vi "NML Bus Scan Sig Recovery 7265.vi"(3 "error in (no error)":errorcluster, 4 "String Read In":string, 5 "VISA Session":refnum<visa-resource-name>) -> (0 "error out":errorcluster, 1 "String Read Out":string, 2 "VISA Session Out":refnum<visa-resource-name>)   [LabVIEW 2021]
uses:
  <vilib>/regexp/Match Regular Expression.xnode
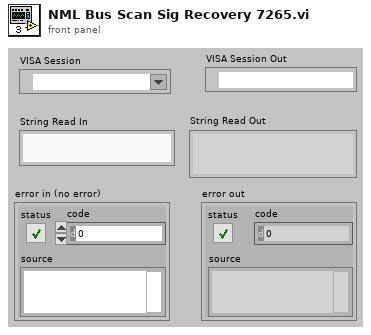
[diagram p1: front panel]
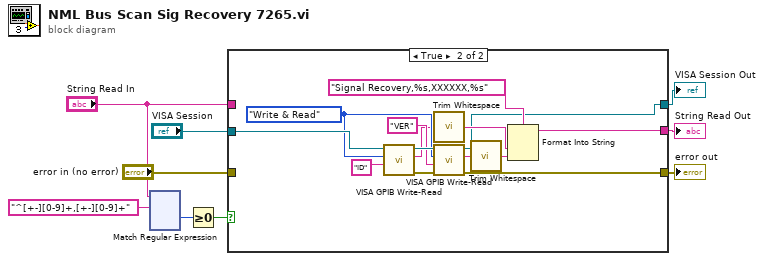
[diagram p0: block diagram]
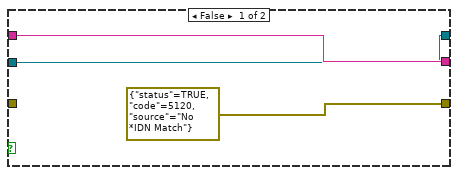
[diagram p2: hidden frame]
diagram:
  n1 = xnode "Match Regular Expression"("input string"="String Read In", "regular expression"="^[+-][0-9]+,[+-][0-9]+") -> ("offset past match"=w4:i32)  [unwired: 4 in, 4 out]
  n2 = Greater Or Equal To 0?(x=w4) -> (x >= 0?=w1:bool)
  n3 = case shown="True" w1 {
    tunnel: [errorcluster {"status"=TRUE, "code"=5120, "source"="No *IDN Match"} ("error out") w13] -> w9
    tunnel: [w12 w24] -> w8
    tunnel: [w11 w14] -> w7
    tunnel: "VISA Session" -> [w11 w23]
    tunnel: "String Read In" -> [w12 _]
    tunnel: "error in (no error)" -> [_ _]
    frame False {
    }
    frame True {
      w21 = enum16{"Write", "Read", "Write & Read"}."Write & Read" ("Action")
      n4 = call "VISA GPIB Write-Read.vi"("Command"="ID" ("String to Write"), "Action"=w21, "VISA resource name"=w23) -> ("error out"=w17:errorcluster, "String Returned"=w19:string, "dup VISA Session"=w22:refnum<visa-resource-name>)  [unwired: 5 in, 1 out]
      n5 = call <vilib>:"Trim Whitespace.vi"("string"=w19) -> ("trimmed string"=w16:string)  [unwired: 1 in]
      n6 = call "VISA GPIB Write-Read.vi"("error in (no error)"=w17, "Command"="VER" ("String to Write"), "Action"=w21, "VISA resource name"=w22) -> ("error out"=w13:errorcluster, "String Returned"=w18:string, "dup VISA Session"=w14:refnum<visa-resource-name>)  [unwired: 4 in, 1 out]
      n7 = call <vilib>:"Trim Whitespace.vi"("string"=w18) -> ("trimmed string"=w15:string)  [unwired: 1 in]
      n8 = Format Into String(format string="Signal Recovery,%s,XXXXXX,%s", w16, w15) -> (resulting string=w24:string)  [unwired: 2 in, 1 out]
    }
  }
  "error out" <- w9
  "String Read Out" <- w8
  "VISA Session Out" <- w7
